vi "RT_Rotation_Integration (SubVI).vi"(1 "W_b(i) [rad/s]":dbl[](array[numeric]), 2 "ang_acc [rad/s^2]":dbl[](array[numeric]), 3 "D_NB":dbl[][](array[numeric]), 4 "q(i) in":dbl[](array[numeric]), 7 "dt":dbl, 9 "dt*0.5":dbl) -> (14 "W(i+1)":dbl[](array[numeric]), 16 "W_b(i+1) [rad/s]":dbl[](array[numeric]), 17 "q(i+1)":dbl[](array[numeric]), 19 "angles (i+1) [rad]":dbl[](array[numeric]))   [LabVIEW 2011]
uses:
  <vilib>/Analysis/_algsub.llb/Vector Norm Type.ctl
  <vilib>/Analysis/coordinate.llb/Euler Rotation Order.ctl
  <vilib>/Analysis/Matrix/Numeric/Conversions/Array To Matrix - RA.vi
  <vilib>/Analysis/Matrix/Numeric/Conversions/Array To Matrix - RA2.vi
  <vilib>/Analysis/baseanly.llb/Real A x B.vi
  <vilib>/Analysis/Matrix/Numeric/Conversions/Matrix To Array - RM.vi
  <vilib>/Analysis/_algsub.llb/Real Vector Norm.vi
  <vilib>/Analysis/Matrix/NI_Matrix.lvlib
  <vilib>/Analysis/NI_AALBase.lvlib
  <vilib>/Analysis/NI_AALPro.lvlib
panel:
  out "Exp_Omega_k_T":dbl[][](array[numeric])
  out "S":dbl[][](array[numeric])
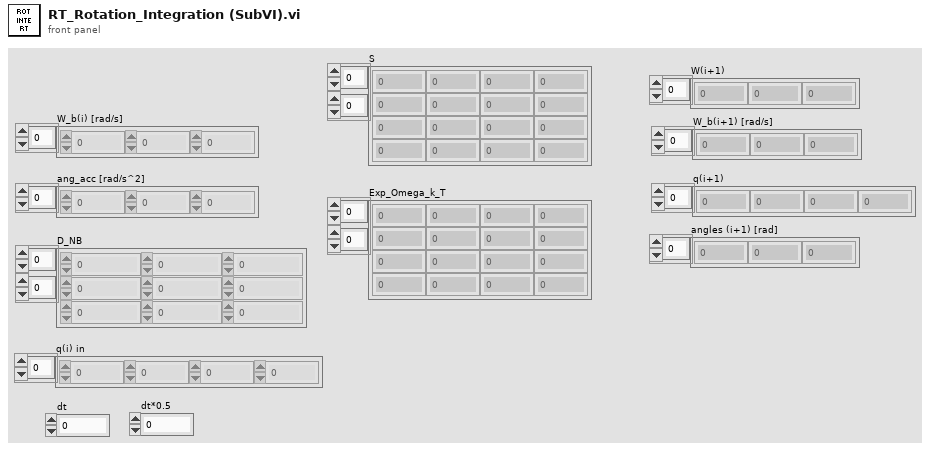
[diagram p1: front panel]
types:
  T1 = typedef "NI_AALPro.lvlib/Euler Rotation Order.ctl" = u16
  T2 = typedef "NI_AALPro.lvlib/Vector Norm Type.ctl" = u16
  T3 = typedef "NI_Matrix.lvlib/RealMatrix.ctl" = dbl[][]
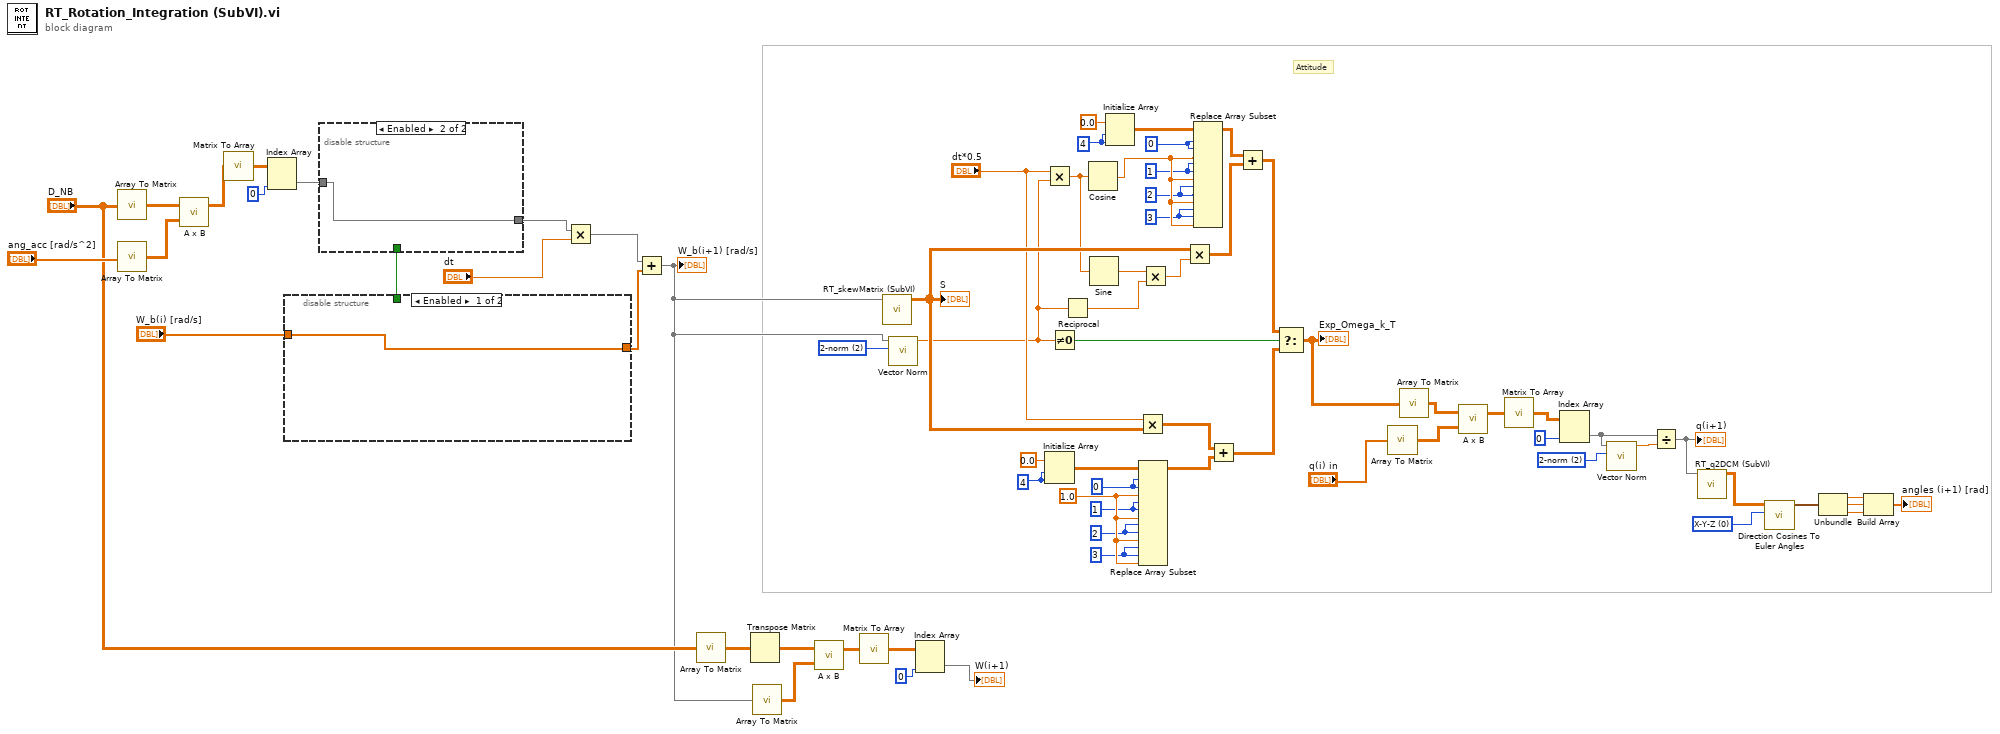
[diagram p0: block diagram]
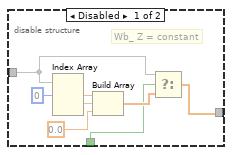
[diagram p2: hidden frame]
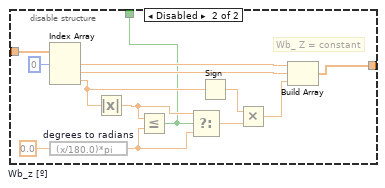
[diagram p3: hidden frame]
diagram:
  w22 = T1 0 items=["X-Y-Z", "X-Z-Y", "Y-X-Z", "Y-Z-X", "Z-X-Y", "Z-Y-X", "X-Y-X", "X-Z-X", "Y-X-Y", "Y-Z-Y", "Z-X-Z", "Z-Y-Z"] ("rotation order")
  w69 = T2 2 items=["1-norm"=1, "2-norm"=2, "Inf-norm"=3, "-Inf-norm"=4, "User Defined"=5] ("norm type")
  w57 = 1.0 ("new element/subarray")
  w52 = 3 ("disabled index (row)")
  w51 = 2 ("disabled index (row)")
  w50 = 1 ("disabled index (row)")
  w53 = 0 ("disabled index (row)")
  w56 = 4 ("dimension size")
  w45 = 3 ("disabled index (row)")
  w46 = 2 ("disabled index (row)")
  w47 = 1 ("disabled index (row)")
  w44 = 0 ("disabled index (row)")
  w34 = 4 ("dimension size")
  w32 = T2 2 items=["1-norm"=1, "2-norm"=2, "Inf-norm"=3, "-Inf-norm"=4, "User Defined"=5] ("norm type")
  # "Attitude"
  n1 = call-poly <vilib>:"Array To Matrix.vi"("Real 2D Array"="D_NB") -> ("Real Matrix"=w30:T3)
  n2 = call-poly <vilib>:"Array To Matrix.vi"("Real 1D Array"="ang_acc [rad/s^2]") -> ("Real Matrix (Column Vector)"=w29:T3)
  n3 = call-poly <vilib>:"A x B.vi"("B"=w29, "A"=w30) -> ("A x B"=w27:T3)  [unwired: 1 out]
  n4 = call-poly <vilib>:"Matrix To Array.vi"("Real Matrix"=w27) -> ("Real 2D Array"=w28:dbl[][])
  n5 = Index Array(array=w28, index (col)=0 ("index (row)")) -> (element=w3:dbl[])  [unwired: 1 in]
  n6 = disable-structure shown="Enabled" {
    disable-tunnel: [w72 w81] -> w4
    disable-tunnel: "W_b(i) [rad/s]" -> [w72 w84]
    disable-tunnel: [_ w73] -> w1
    frame Enabled {
    }
    frame Disabled {
      w80 = 0.0  # Wb_z [º]
      # "Wb_ Z = constant"
      n7 = Index Array(array=w84, index #1=0 ("index")) -> (element #1=w83:dbl, element #2=w82:dbl, element #3=w76:dbl)  [unwired: 2 in]
      n8 = expression code="(x/180.0)*pi" "degrees to radians"(w80) -> (w79:dbl)
      n9 = Absolute Value(x=w76) -> (abs(x)=w78:dbl)
      n10 = Less Or Equal?(x=w78, y=w79) -> (x <= y?=w73:bool)
      n11 = Select(t=w78, s=w73, f=w79) -> (s? t:f=w77:dbl)
      n12 = Sign(1:w76) -> (0:w75:dbl)
      n13 = Multiply(x=w75, y=w77) -> (x*y=w74:dbl)
      n14 = Build Array(w83, w82, w74) -> (w81:dbl[])
    }
  }
  n15 = disable-structure shown="Enabled" {
    disable-tunnel: w3 -> [w89 w94]
    disable-tunnel: [w87 w94] -> w2
    disable-tunnel: w1 -> [w86 _]
    frame Disabled {
      # "Wb_ Z = constant"
      n16 = Index Array(array=w89, index #1=0 ("index")) -> (element #1=w92:dbl, element #2=w91:dbl)  [unwired: 2 in, 1 out]
      n17 = Build Array(w92, w91, 0.0 ("element")) -> (w88:dbl[])
      n18 = Select(t=w89, s=w86, f=w88) -> (s? t:f=w87:dbl[])
    }
    frame Enabled {
    }
  }
  n19 = Multiply(x=w2, y="dt") -> (x*y=w23:dbl[])
  n20 = Add(x=w23, y=w4) -> (x+y=w7:dbl[])
  "W_b(i+1) [rad/s]" <- w7
  n21 = call-poly <vilib>:"Array To Matrix.vi"("Real 2D Array"="D_NB") -> ("Real Matrix"=w9:T3)
  n22 = Transpose Matrix(1:w9) -> (0:w10:T3)
  n23 = call-poly <vilib>:"Array To Matrix.vi"("Real 1D Array"=w7) -> ("Real Matrix (Column Vector)"=w11:T3)
  n24 = call-poly <vilib>:"A x B.vi"("B"=w11, "A"=w10) -> ("A x B"=w13:T3)  [unwired: 1 out]
  n25 = call-poly <vilib>:"Matrix To Array.vi"("Real Matrix"=w13) -> ("Real 2D Array"=w12:dbl[][])
  n26 = call "RT_skewMatrix (SubVI).vi"("vector"=w7) -> ("skew matrix"=w59:dbl[][])  [unwired: 10 in]
  "S" <- w59
  n27 = call-poly <vilib>:"Vector Norm.vi"("norm type"=w32, "Input Vector"=w7) -> ("norm"=w37:dbl)  [unwired: 8 in, 1 out]
  n28 = Index Array(array=w12, index (col)=0 ("index (row)")) -> (element=→"W(i+1)":dbl[])  [unwired: 1 in]
  n29 = Multiply(x="dt*0.5", y=w37) -> (x*y=w36:dbl)
  n30 = Initialize Array(0.0 ("element"), w56, w56) -> (w54:dbl[][])
  n31 = Not Equal To 0?(x=w37) -> (x != 0?=w33:bool)
  n32 = Reciprocal(x=w37) -> (1/x=w39:dbl)
  n33 = Cosine(x=w36) -> (cos(x)=w48:dbl)
  n34 = Sine(x=w36) -> (sin(x)=w38:dbl)
  n35 = Initialize Array(0.0 ("element"), w34, w34) -> (w42:dbl[][])
  n36 = Multiply(x="dt*0.5", y=w59) -> (x*y=w60:dbl[][])
  n37 = Replace Array Subset(array=w54, new element #1=w57, index (row) #1=w53, index (col) #1=w53, new element #2=w57, index (row) #2=w50, index (col) #2=w50, new element #3=w57, index (row) #3=w51, index (col) #3=w51, new element #4=w57, index (row) #4=w52, index (col) #4=w52) -> (w61:dbl[][])
  n38 = Multiply(x=w38, y=w39) -> (x*y=w40:dbl)
  n39 = Multiply(x=w59, y=w40) -> (x*y=w41:dbl[][])
  n40 = Replace Array Subset(array=w42, new element #1=w48, index (row) #1=w44, index (col) #1=w44, new element #2=w48, index (row) #2=w47, index (col) #2=w47, new element #3=w48, index (row) #3=w46, index (col) #3=w46, new element #4=w48, index (row) #4=w45, index (col) #4=w45) -> (w43:dbl[][])
  n41 = Add ("Add.vi")(x=w60, y=w61) -> (x+y=w62:dbl[][])
  n42 = Add ("Add.vi")(x=w43, y=w41) -> (x+y=w49:dbl[][])
  n43 = Select(t=w49, s=w33, f=w62) -> (s? t:f=w68:dbl[][])
  "Exp_Omega_k_T" <- w68
  n44 = call-poly <vilib>:"Array To Matrix.vi"("Real 1D Array"="q(i) in") -> ("Real Matrix (Column Vector)"=w66:T3)
  n45 = call-poly <vilib>:"Array To Matrix.vi"("Real 2D Array"=w68) -> ("Real Matrix"=w67:T3)
  n46 = call-poly <vilib>:"A x B.vi"("B"=w66, "A"=w67) -> ("A x B"=w64:T3)  [unwired: 1 out]
  n47 = call-poly <vilib>:"Matrix To Array.vi"("Real Matrix"=w64) -> ("Real 2D Array"=w65:dbl[][])
  n48 = Index Array(array=w65, index (col)=0 ("index (row)")) -> (element=w71:dbl[])  [unwired: 1 in]
  n49 = call-poly <vilib>:"Vector Norm.vi"("norm type"=w69, "Input Vector"=w71) -> ("norm"=w70:dbl)  [unwired: 8 in, 1 out]
  n50 = Divide(x=w71, y=w70) -> (x/y=w17:dbl[])
  "q(i+1)" <- w17
  n51 = call "RT_q2DCM (SubVI).vi"("Quaternion"=w17) -> ("DCM"=w16:dbl[][])  [unwired: 10 in]
  n52 = call <vilib>:"Direction Cosines To Euler Angles.vi"("rotation order"=w22, "Direction Cosines"=w16) -> ("Euler Angles"=w19:cluster{"phi":dbl, "theta":dbl, "psi":dbl})  [unwired: 8 in, 1 out]
  n53 = Unbundle(w19) -> ("phi"=w21:dbl, "theta"=w20:dbl, "psi"=w18:dbl)
  n54 = Build Array(w21, w20, w18) -> (→"angles (i+1) [rad]":dbl[])
